vi "Configure List Sweep_.vi"(5 "Sweep Function A (0: Frequency)":u16(ring) items=["Frequency", "Voltage", "Current", "Bias Voltage", "Bias Current", "DC Source Voltage"], 7 "Sweep Function B (0: None)":u16(ring) items=["None", "Impedance Range", "Frequency", "Voltage", "Current", "Bias Voltage", "Bias Current", "DC Source Voltage"], 8 "error in (no error)":errorcluster, 9 "Sweep Mode (0: Sequence)":u16(ring) items=["Sequence", "Stepped"], 10 "Sweep Point Array":dbl[](array[numeric])=[0.0, 0.0, 0.0, 0.0, 0.0], 11 "Agilent E4980 in":refnum<class "Agilent E4980.lvclass">) -> (0 "error out":errorcluster, 3 "Agilent E4980 out":refnum<class "Agilent E4980.lvclass">)   [LabVIEW 2020, in "Agilent E4980.lvclass"]
uses:
  Agilent E4980.lvclass
  C:/Sandbox/RF Bench/Source Code/WiSpry Test Framework/Instruments/Instrument.lvclass
  Instrument.lvclass/Instrument.ctl
  <instrlib>/Agilent E4980/Agilent E4980.lvlib
  Instrument.lvclass
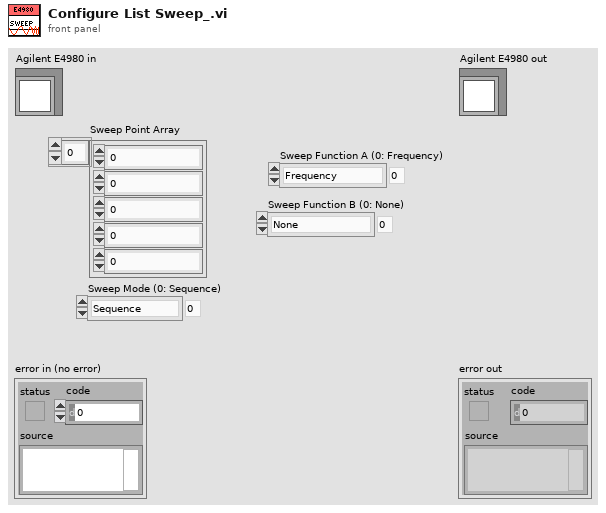
[diagram p1: front panel]
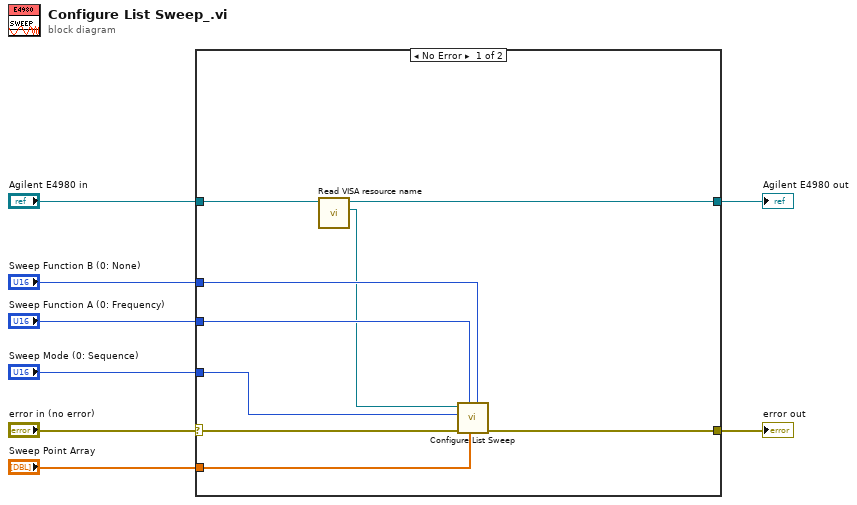
[diagram p0: block diagram]
diagram:
  n1 = case shown="No Error" "error in (no error)" {
    selector: "error in (no error)" -> [w17 w19]
    tunnel: [w16 w19] -> w7
    tunnel: [w10 w18] -> w6
    tunnel: "Agilent E4980 in" -> [w11 w18]
    tunnel: "Sweep Function A (0: Frequency)" -> [w15 _]
    tunnel: "Sweep Function B (0: None)" -> [w14 _]
    tunnel: "Sweep Mode (0: Sequence)" -> [w13 _]
    tunnel: "Sweep Point Array" -> [w12 _]
    frame No Error {
      n2 = call "Read VISA resource name.vi"("Instrument in"=w11) -> ("VISA resource name"=w9:refnum<visa-resource-name>, "Instrument out"=w10:refnum<class "Agilent E4980.lvclass">)  [unwired: 9 in]
      n3 = call <instrlib>:"Configure List Sweep.vi"("Sweep Function B (0: None)"=w14, "Sweep Point Array"=w12, "Sweep Function A (0: Frequency)"=w15, "error in (no error)"=w17, "Sweep Mode (0: Sequence)"=w13, "VISA resource name"=w9) -> ("error out"=w16:errorcluster)  [unwired: 5 out]
    }
    frame Error {
    }
  }
  "error out" <- w7
  "Agilent E4980 out" <- w6
